vi "Dispose.vi"(8 "error in":errorcluster, 11 "NYStyleVeggiePizza":refnum<class "NYStyleVeggiePizza.lvclass">) -> (0 "error out":errorcluster)   [LabVIEW 2020, in "FactoryMethod.lvlib" / "PizzaFactoryMethod.lvlib" / "NYStyleVeggiePizza.lvclass"]
uses:
  NYStyleVeggiePizza.lvclass
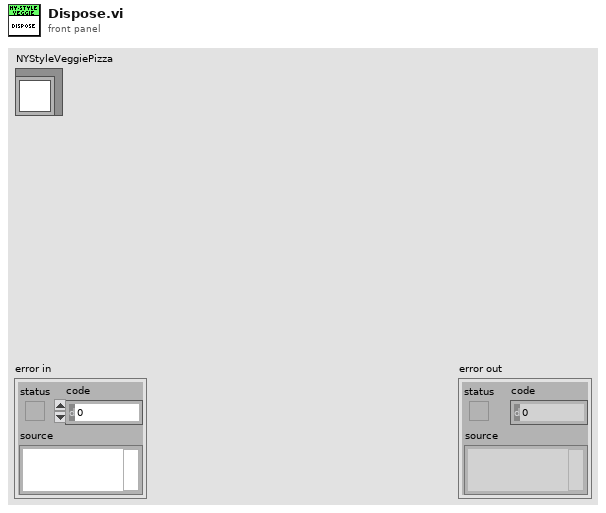
[diagram p1: front panel]
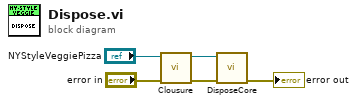
[diagram p0: block diagram]
diagram:
  n1 = call-dynamic "Clousure.vi"("error in"="error in", "NYStyleVeggiePizza"="NYStyleVeggiePizza") -> ("error out"=w3:errorcluster, "NYStyleVeggiePizza"=w4:refnum<class "NYStyleVeggiePizza.lvclass">)  [unwired: 8 in]
  n2 = call-dynamic "DisposeCore.vi"("error in (no error)"=w3, "NYStyleVeggiePizza"=w4) -> ("error out"=→"error out":errorcluster)  [unwired: 8 in, 1 out]
